vi "QuickTest.vi"() -> ()   [LabVIEW 2012]
uses:
  Controls/TestData.ctl
  Classes/Instruments.lvclass
panel:
  in  "Int Time":i32=1
  in  "Is":dbl=0.1
  out "Data Out":T1 {"50mA Data"."Current,mA" format="%_6g"; "50mA Data"."WL" format="%_6g"; "50mA Data"."Voltage" format="%_6g"; "50mA Data"."Power" format="%_6g"; "20mA Data"."Reverse" format="%#_3g"; "20mA Data"."Current,mA" format="%_6g"; "20mA Data"."Knee Current" format="%#_3g"; "20mA Data"."WL" format="%_6g"; "20mA Data"."Voltage" format="%_6g"; "20mA Data"."Power" format="%_5g"}
  out "Graph":cluster{"Wavelength":dbl[], "EL Spectrum":dbl[]}(graph)
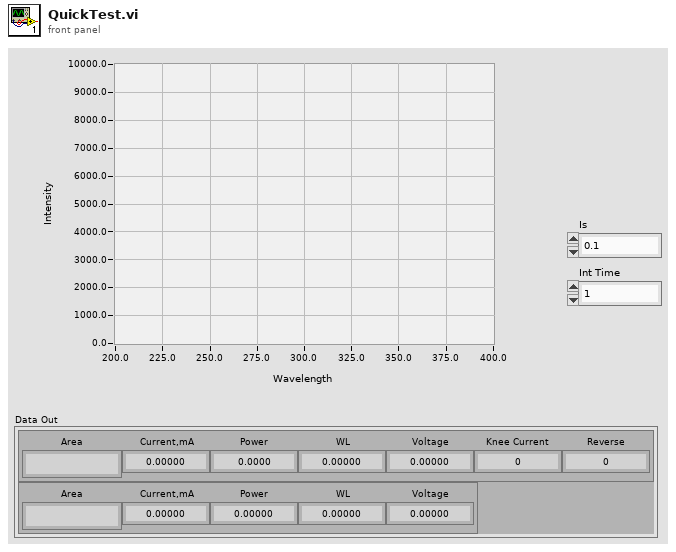
[diagram p1: front panel]
types:
  T1 = typedef "TestData.ctl" = cluster{"20mA Data":cluster{"Area":string, "Current,mA":dbl, "Power":dbl, "WL":dbl, "Voltage":dbl, "Knee Current":dbl, "Reverse":dbl}, "50mA Data":cluster{"Area":string, "Current,mA":dbl, "Power":dbl, "WL":dbl, "Voltage":dbl}}
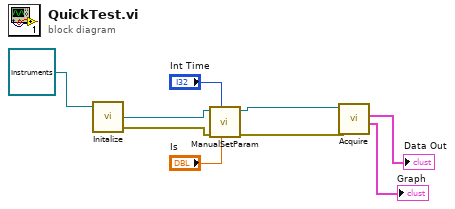
[diagram p0: block diagram]
diagram:
  n1 = call-dynamic "Initalize.vi"("Instruments in"=refnum<class "Instruments.lvclass"> refnum) -> ("error out"=w7:errorcluster, "Instruments out"=w8:refnum<class "Instruments.lvclass">)  [unwired: 3 in]
  n2 = call-dynamic "ManualSetParam.vi"("Is"="Is", "Int Time"="Int Time", "error in (no error)"=w7, "Instruments in"=w8) -> ("error out"=w6:errorcluster, "Instruments out"=w5:refnum<class "Instruments.lvclass">)  [unwired: 6 in]
  n3 = call-dynamic "Acquire.vi"("error in (no error)"=w6, "Instruments in"=w5) -> ("20mA Spectra"=→"Graph":cluster{"Wavelength":dbl[], "EL Spectrum":dbl[]}, "Data Out"=→"Data Out":T1)  [unwired: 4 in, 4 out]
